vi "Test Guards.vi"(6 "Data":T2, 11 "Guard":T1) -> (0 "error out":errorcluster, 3 "pass guard?":bool)   [LabVIEW 2019, in "LVCOOOP Tests.lvlib" / "State Machine API.lvlib"]
uses:
  State Machine API.lvlib
  types/Data.ctl
  types/Guard.ctl
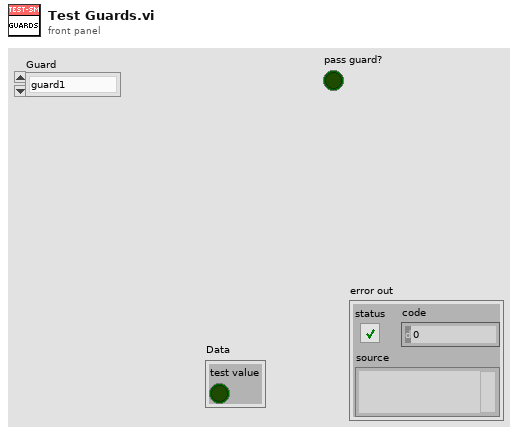
[diagram p1: front panel]
types:
  T1 = typedef "LVCOOOP Tests.lvlib/State Machine API.lvlib/Guard.ctl" = enum16{"guard1"}
  T2 = typedef "LVCOOOP Tests.lvlib/State Machine API.lvlib/Data.ctl" = cluster{"test value":bool}
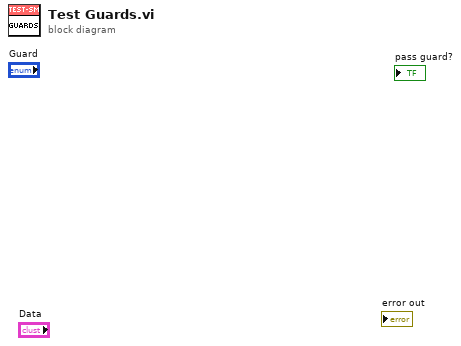
[diagram p0: block diagram]
diagram:
